vi "DBC Get Msg Publisher.vi"(9 "pPublisher":string, 10 "pMsgName":string, 11 "DBCHandle":u64) -> (1 "pPublisher out":string, 2 "pMsgName out":string, 3 "function return":i32)   [LabVIEW 2010, in "dbc_parser.lvlib"]
doc: "int WINAPI DBC_GetMsgPublisher(long long DBCHandle, char* pMsgName, char* pPublisher);"
uses:
  dbc_parser.lvlib
  USB2XXX/trunk/USB2XXX/USB2XXX/vs2019/Release/USB2XXX.dll
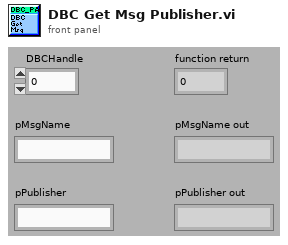
[diagram p1: front panel]
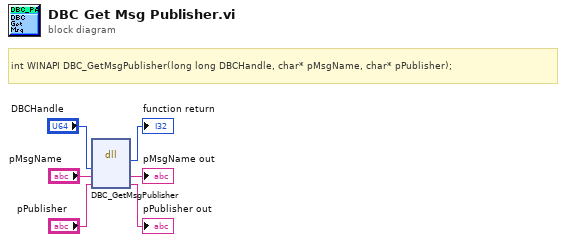
[diagram p0: block diagram]
diagram:
  # "int WINAPI DBC_GetMsgPublisher(long long DBCHandle, char* pMsgName, char* pPublisher);"
  n1 = dll-call lib="E:/Projects/USB2XXX/trunk/USB2XXX/USB2XXX/vs2019/Release/USB2XXX.*" fn="DBC_GetMsgPublisher"("DBCHandle"="DBCHandle", "pMsgName"="pMsgName", "pPublisher"="pPublisher") -> (→"function return":i32, "pMsgName"=→"pMsgName out":string, "pPublisher"=→"pPublisher out":string)  [unwired: 4 in, 2 out]
